vi "Not Found Error.vi"(8 "error in (no error)":errorcluster, 9 "additional info":string, 11 "item type":string) -> (0 "error out":errorcluster)   [LabVIEW 2013, in "i3-json.lvlib"]
uses:
  i3-json.lvlib
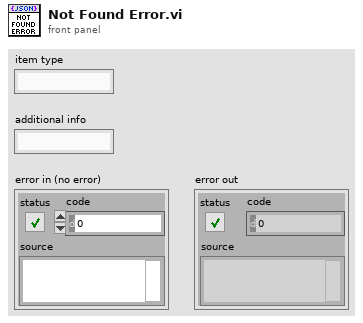
[diagram p1: front panel]
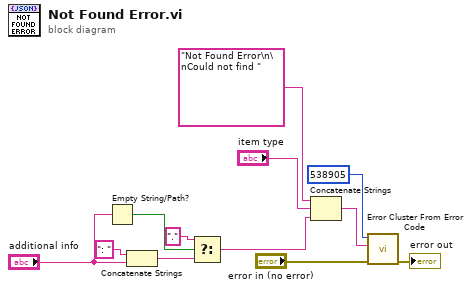
[diagram p0: block diagram]
diagram:
  n1 = Empty String/Path?(string/path="additional info") -> (empty?=w6:bool)
  n2 = Concatenate Strings(": " ("string"), "additional info") -> (w2:string)
  n3 = Select(t="." ("datatype"), s=w6, f=w2) -> (s? t:f=w1:string)
  n4 = Concatenate Strings("Not Found Error\n\nCould not find " ("error message (\"\")"), "item type", w1) -> (w9:string)
  n5 = call <vilib>:"Error Cluster From Error Code.vi"("error in (no error)"="error in (no error)", "error message (\"\")"=w9, "error code (0)"=538905) -> ("error out"=→"error out":errorcluster)  [unwired: 6 in]
